vi "fotoncounter+lockin+fastratio_LV2010.vi"() -> ()   [LabVIEW 2010]
uses:
  Instance          14 40Saved   fotoncounter+lockin+fastratio v1 .vi
  Instance          13 40Saved   fotoncounter+lockin+fastratio v1 .vi
  Instance          33 40Saved   fotoncounter+lockin+fastratio v1 .vi
  Instance           2 40Saved   fotoncounter+lockin+fastratio v1 .vi
  Instance           5 40Saved   fotoncounter+lockin+fastratio v1 .vi
  Instance           6 40Saved   fotoncounter+lockin+fastratio v1 .vi
  Instance           7 40Saved   fotoncounter+lockin+fastratio v1 .vi
  Instance          15 40Saved   fotoncounter+lockin+fastratio v1 .vi
  Instance           8 40Saved   fotoncounter+lockin+fastratio v1 .vi
  Instance           9 40Saved   fotoncounter+lockin+fastratio v1 .vi
  Instance          10 40Saved   fotoncounter+lockin+fastratio v1 .vi
  Instance          11 40Saved   fotoncounter+lockin+fastratio v1 .vi
  Instance           1 40Saved   fotoncounter+lockin+fastratio v1 .vi
  Instance          18 40Saved   fotoncounter+lockin+fastratio v1 .vi
  Instance          19 40Saved   fotoncounter+lockin+fastratio v1 .vi
  Instance          23 40Saved   fotoncounter+lockin+fastratio v1 .vi
  Instance          17 40Saved   fotoncounter+lockin+fastratio v1 .vi
  Instance          22 40Saved   fotoncounter+lockin+fastratio v1 .vi
  Instance          20 40Saved   fotoncounter+lockin+fastratio v1 .vi
  Instance          21 40Saved   fotoncounter+lockin+fastratio v1 .vi
  Instance          26 40Saved   fotoncounter+lockin+fastratio v1 .vi
  Instance          27 40Saved   fotoncounter+lockin+fastratio v1 .vi
  Instance          29 40Saved   fotoncounter+lockin+fastratio v1 .vi
  <vilib>/Utility/file.llb/Write To Spreadsheet File (DBL).vi
  Instance          24 40Saved   fotoncounter+lockin+fastratio v1 .vi
  <vilib>/Utility/file.llb/Read From Spreadsheet File (DBL).vi
  Instance          32 40Saved   fotoncounter+lockin+fastratio v1 .vi
  Instance          31 40Saved   fotoncounter+lockin+fastratio v1 .vi
  Instance          30 40Saved   fotoncounter+lockin+fastratio v1 .vi
panel:
  out "lockin corrected count":cluster{dbl[], dbl[]}(graph)
  in  "Array":dbl[](array[numeric])
  in  "Lockin settings":T1={"slope"=1, "Input Mode"=0, "time constant"=6, "display type"=1, "Range"=7, "Line reject"=1, "Filter Type"=0, "Auto freq tuning"=TRUE, "Filter Frequency (Hz)"=1000.0, "Auto Sensitivity"=FALSE, "Auto Measure"=FALSE, "Auto Phase"=TRUE} {"Filter Frequency (Hz)" min=2.0 max=1250000.0 step=1.0; "Filter Type" items=["Flat", "Notch", "Low-Pass", "Bandpass"]; "Line reject" items=["OFF", "2F", "F", "F & 2F"]; "Range" items=["100 nV", "300 nV", "1 uV", "3 uV", "10 uV", "30 uV", "100 uV", "300 uV", "1 mV", "3 mV", "10 mV", "30 mV", "100 mV", "300 mV", "1 V", "3 V"]; "display type" items=["Output %", "Output calibrated ", "Ratio", "log Ratio", "ADC 1", "ADC 2", " ADC 3", "ADC 4", "Noise %", "Noise Calibrated", "Ref. Frequency"]; "time constant" items=["1 ms", "3 ms", "10 ms", "30 ms", "100 ms", "300 ms", "1 s", "3 s", "10 s", "30 s", "100 s", "300 s", "1 ks", "3 ks"]; "Input Mode" items=["Voltage Input ( A or A-B)", "Current Input 10E6 V/A", "Current Input 10E8 V/A"]; "slope" items=["6dB/octave", "12dB/octave"]}
  in  "Cluster":T2={"slope"=1, "Input Mode"=0, "time constant"=0, "display type"=1, "Range"=13} {"Range" items=["100 nV", "300 nV", "1 uV", "3 uV", "10 uV", "30 uV", "100 uV", "300 uV", "1 mV", "3 mV", "10 mV", "30 mV", "100 mV", "300 mV", "1 V", "3 V"]; "display type" items=["Output %", "Output calibrated ", "Ratio", "log Ratio", "ADC 1", "ADC 2", " ADC 3", "ADC 4", "Noise %", "Noise Calibrated", "Ref. Frequency"]; "time constant" items=["1 ms", "3 ms", "10 ms", "30 ms", "100 ms", "300 ms", "1 s", "3 s", "10 s", "30 s", "100 s", "300 s", "1 ks", "3 ks"]; "Input Mode" items=["Voltage Input ( A or A-B)", "Current Input 10E6 V/A", "Current Input 10E8 V/A"]; "slope" items=["6dB/octave", "12dB/octave"]}
  out "lockin":i32
  out "counter B":i32=147
  out "counter A":i32=5821
  out "LOCKIN OUTPUT DATA":cluster{"Y":dbl[], "Y":dbl[]}[](graph)=[{"Y"=[1.0], "Y"=[0.08234234]}]
  in  "EG&G 5209\nlockin amplifier\nGPIB address":u8=12 min=1 max=32 step=1
  out "# count periods done":i32=1
  out "Data Bit value":i32=1
  out "PHOTON COUNTER DATA":cluster{"all rows":dbl[], "all rows":dbl[]}[](graph)=[{"all rows"=[1.0], "all rows"=[5821.0]}, {"all rows"=[1.0], "all rows"=[147.0]}]
  in  "T select":i16(slide) scale=0.0..2.0
  in  "A scan step (V)":ext=-0.005 format="%.3e"
  in  "B scan step(V)":ext=-0.005 format="%.3e"
  in  "T scan step (V)":ext=0.02 format="%.3e"
  out "error 7":bool
  in  "A mode":bool=TRUE
  in  "B mode":bool=TRUE
  in  "T mode":bool=TRUE
  in  "A level (V)":ext=0.028 format="%.3e"
  in  "B level (V)":ext=0.028 format="%.3e"
  in  "T level (V)":ext=-0.01 format="%.3e"
  in  "B Preset":ext=1.0
  in  "count mode":i16(slide) scale=0.0..3.0 scale format="%.2f"
  in  "Path":path=path "C:/lvtemp/phototemp"
  out "error 6":bool
  in  "A slope":bool=TRUE
  in  "B slope":bool=TRUE
  in  "T slope":bool
  in  "trigger slope":bool
  out "error 5":bool
  in  "trigger level":ext=0.5 format="%.3f"
  in  "A scan step":ext=0.000005 format="%.3e"
  in  "dwell source":i32(slide) scale=0.0..1.0
  in  "dwell time":ext=0.1 format="%.4f"
  in  "# count periods\n(2000 max.)":i32=1
  in  "A select":i16(slide)=1 scale=0.0..1.0
  in  "B select":i16(slide)=1 scale=1.0..2.0 scale format="%.2f"
  in  "SR400\nphoton counter\nGPIB address":string="0:23"
  in  "B gate delay":ext=0.00027000000000000000001 format="%.3e"
  in  "B gate mode":i16(slide)=1 scale=0.0..2.0
  out "error 2":bool
  in  "B gate width":ext=0.00021 format="%.3e"
  in  "B scan step":ext=0.000005 format="%.3e"
  in  "A gate delay":ext=0.00001 format="%.3e"
  in  "A gate mode":i16(slide)=1 scale=0.0..2.0 scale format="%.2f"
  in  "A gate width":ext=0.00021 format="%.3e"
  in  "T Preset":ext=5.0
  # "SR400 PHOTON COUNTER + EG&G 5209 LOCKIN AMPLIFIER"
  # "ADDRESSING/TRIGGER/DWELL SETTINGS"
  # "COUNTER/INPUT SETTINGS"
  # "photon counter GPIB Board 0, address 23\nEG&G lockin GPIB Board 0, address 12"
  # "RISE\n\nFALL"
  # "(s)"
  # "note: valid dwell time\n0.002  to 60.0 s"
  # "(s)"
  # "DISCRIMINATOR SETTINGS"
  # "GATE SETTINGS"
  # "FIXED\n\nSCAN"
  # "RISE\n\nFALL"
  # "RISE\n\nFALL"
  # "FIXED\n\nSCAN"
  # "FIXED\n\nSCAN"
  # "RISE\n\nFALL"
  # "note: valid disc levels \n-0.30 to 0.30 V"
  # "note: valid scan steps \n-0.020 to 0.020 V"
  # "\"...The greatest trick the Devil ever pulled was convincing the world he didn't exist...\" (and then inventing LabView)..."
  # "This makes the lockin work again. no idea if the settings are right, or even need to be messed with"
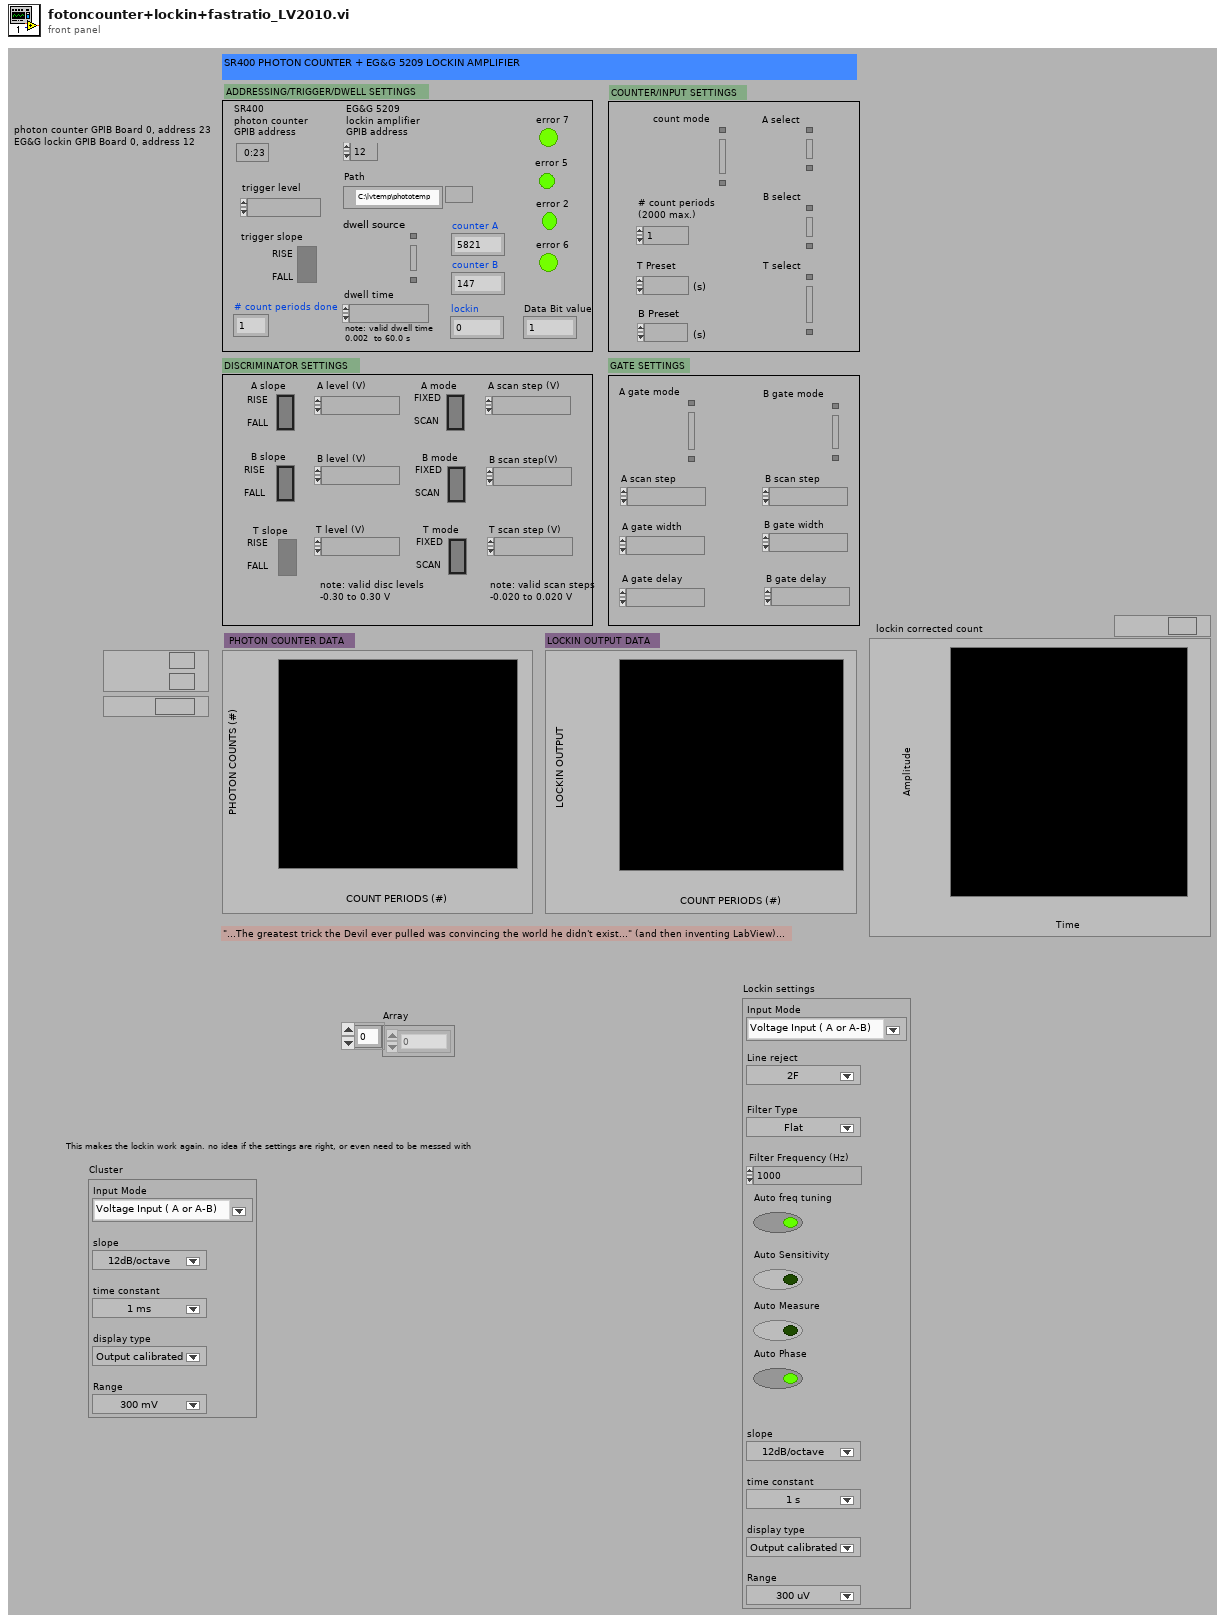
[diagram p1: front panel]
types:
  T1 = cluster{"slope":i32, "Input Mode":i32, "time constant":i32, "display type":i32, "Range":i32, "Line reject":i32, "Filter Type":i32, "Auto freq tuning":bool, "Filter Frequency (Hz)":dbl, "Auto Sensitivity":bool, "Auto Measure":bool, "Auto Phase":bool}
  T2 = cluster{"slope":i32, "Input Mode":i32, "time constant":i32, "display type":i32, "Range":i32}
  T3 = enum16{"open", "open or create", "create or replace", "create", "open (read only)"}
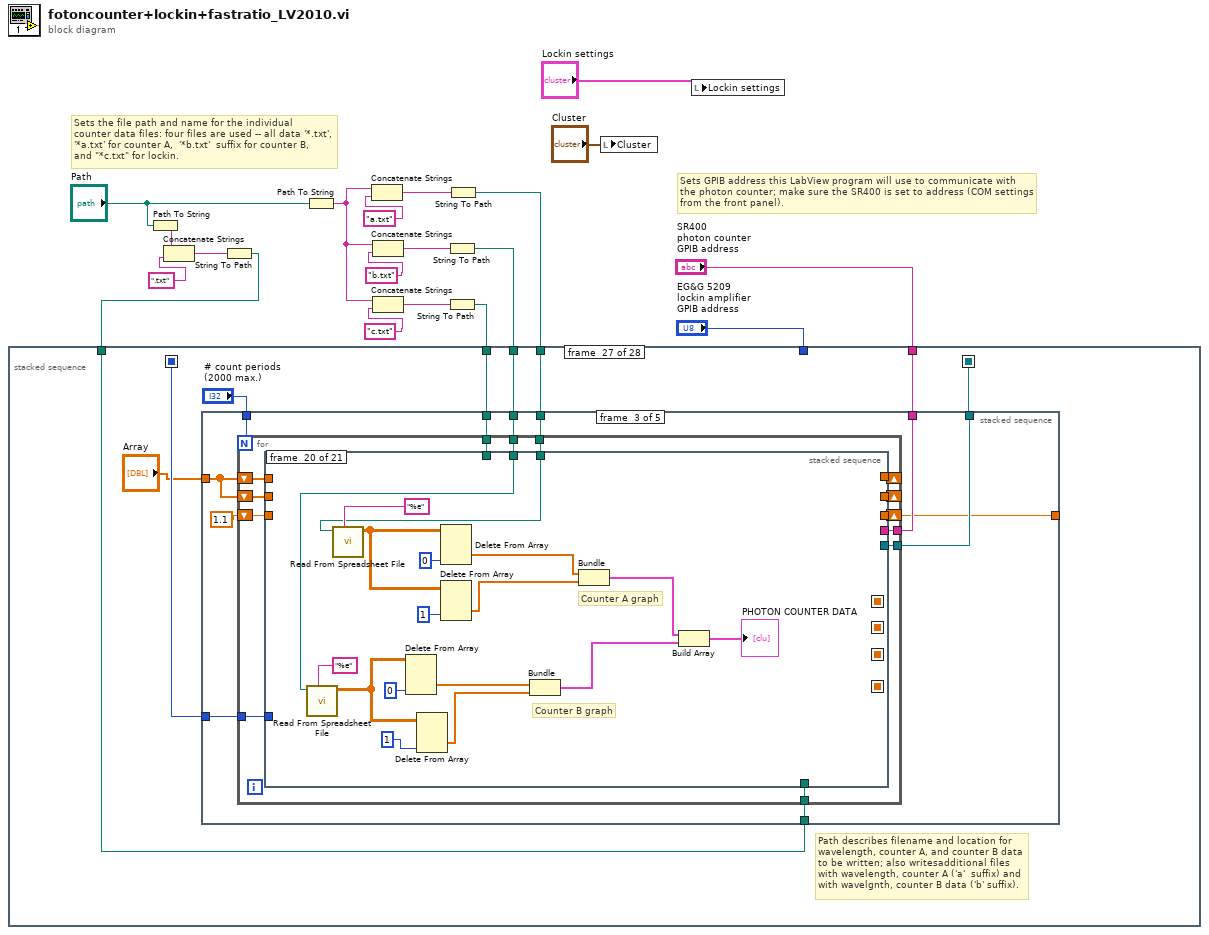
[diagram p0: block diagram]
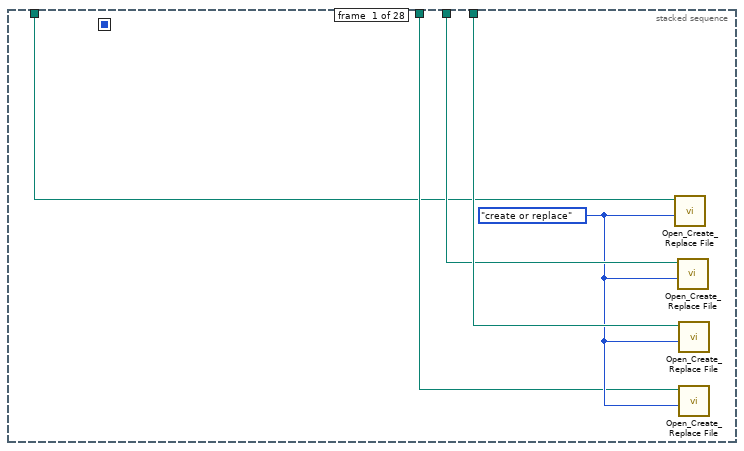
[diagram p2: hidden frame]
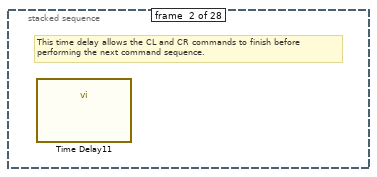
[diagram p3: hidden frame]
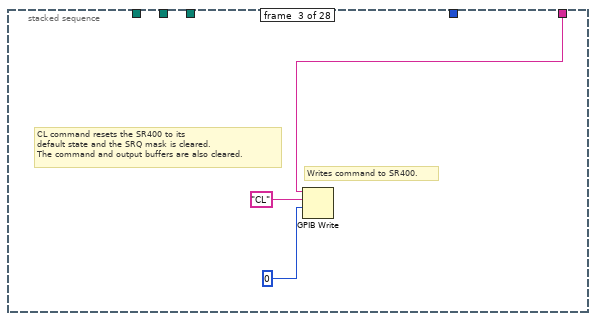
[diagram p4: hidden frame]
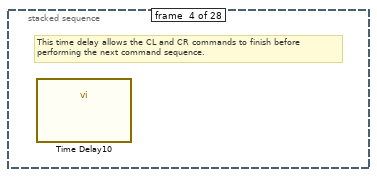
[diagram p5: hidden frame]
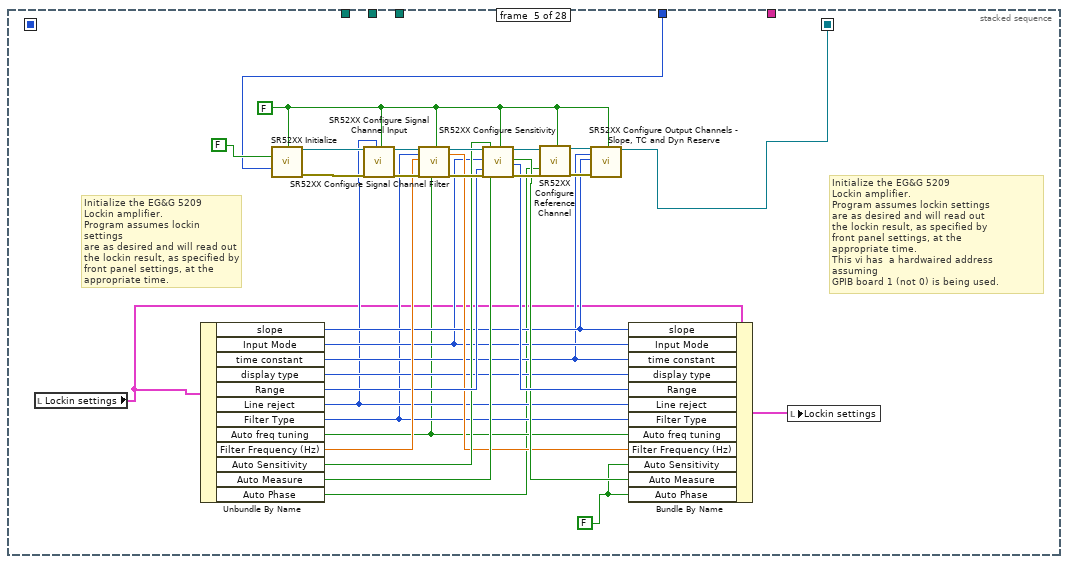
[diagram p6: hidden frame]
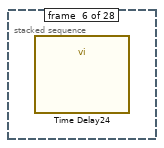
[diagram p7: hidden frame]
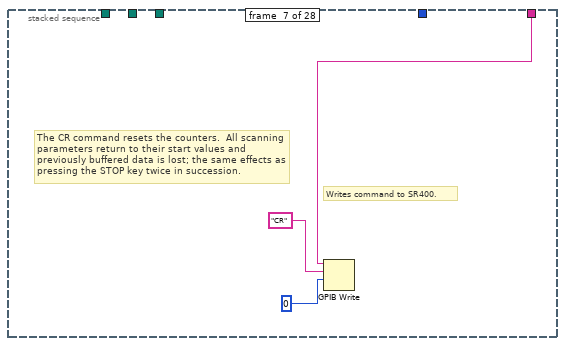
[diagram p8: hidden frame]
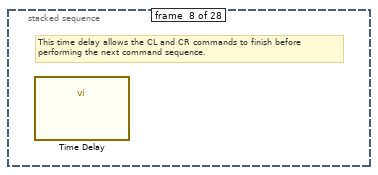
[diagram p9: hidden frame]
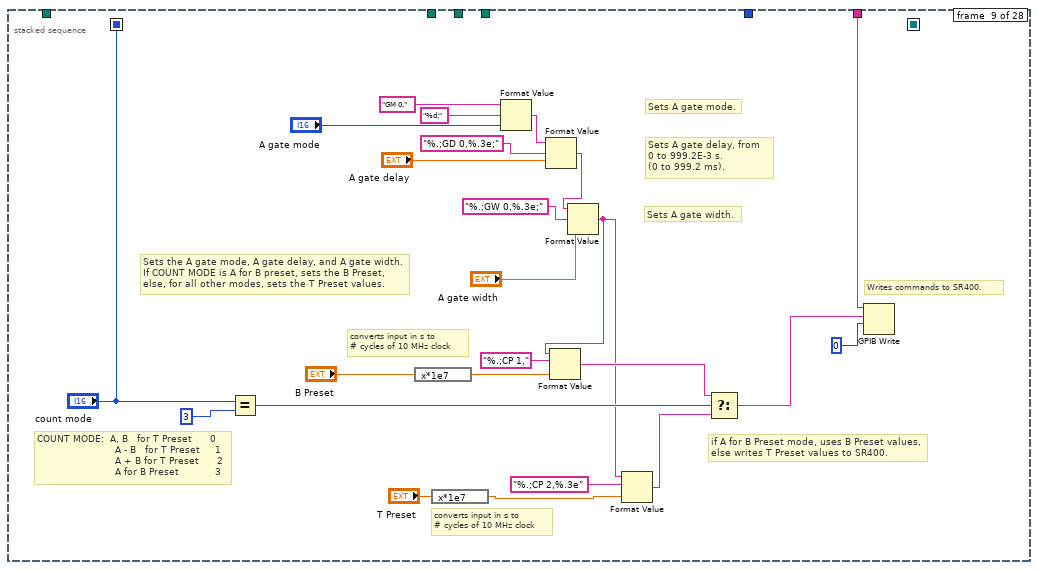
[diagram p10: hidden frame]
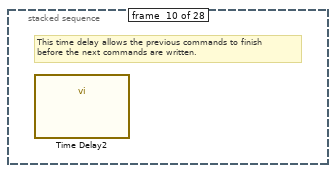
[diagram p11: hidden frame]
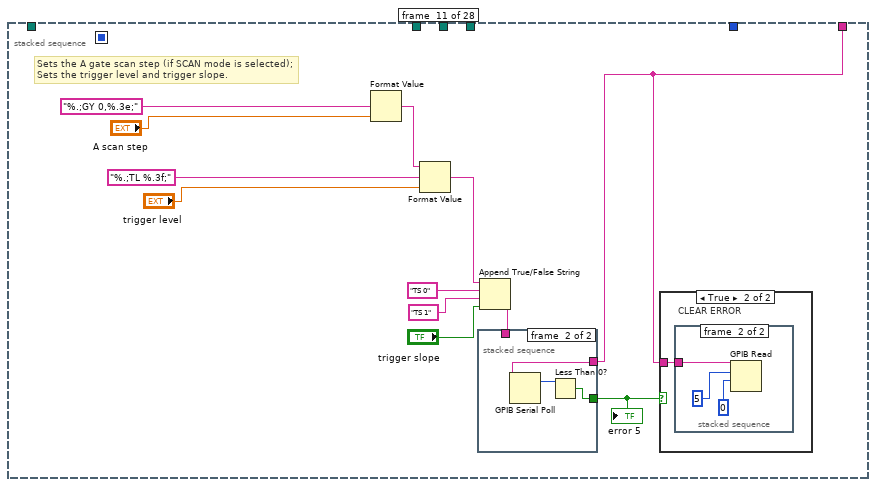
[diagram p12: hidden frame]
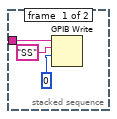
[diagram p14: hidden frame]
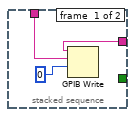
[diagram p15: hidden frame]
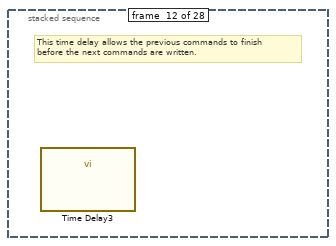
[diagram p16: hidden frame]
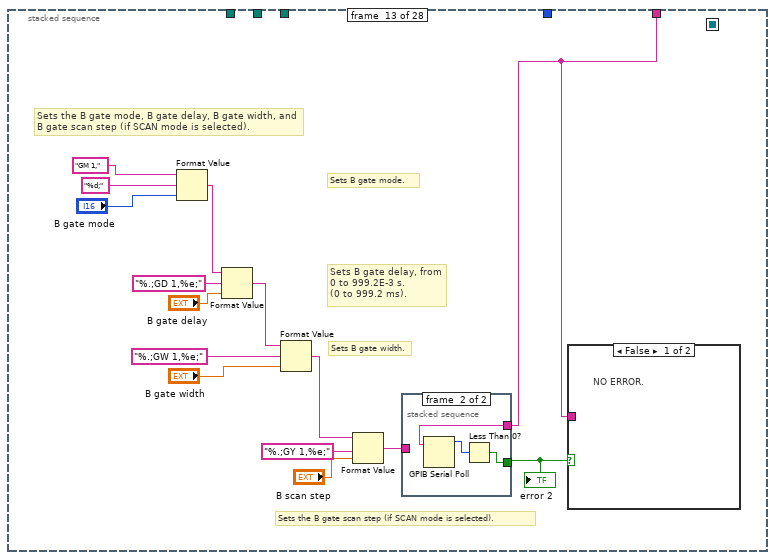
[diagram p17: hidden frame]
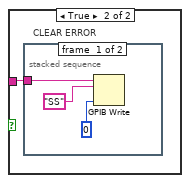
[diagram p18: hidden frame]
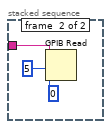
[diagram p19: hidden frame]
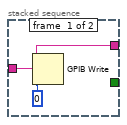
[diagram p20: hidden frame]
diagram:
  # "Sets the file path and name for the individual\ncounter data files: four files are used -- all data '*.txt',\n'*a.txt' for counter A,  '*b.txt'  suffix for counter B,\nand \"*c.txt\" for lockin."
  # "Sets GPIB address this LabView program will use to communicate with\nthe photon counter; make sure the SR400 is set to address (COM settings\nfrom the front panel)."
  n1 = Path To String(path="Path") -> (string=w13:string)
  n2 = Concatenate Strings(w13, ".txt") -> (w11:string)
  n3 = String To Path(string=w11) -> (path=w3:path)
  n4 = Path To String(path="Path") -> (string=w6:string)
  n5 = Concatenate Strings(w6, "a.txt") -> (w14:string)
  n6 = Concatenate Strings(w6, "b.txt") -> (w17:string)
  n7 = Concatenate Strings(w6, "c.txt") -> (w8:string)
  n8 = String To Path(string=w17) -> (path=w15:path)
  n9 = String To Path(string=w8) -> (path=w5:path)
  n10 = String To Path(string=w14) -> (path=w16:path)
  n11 = stacked-sequence {
    seq-local: [_ _ _ _ _ _ _ _ "count mode" _ _ _ _ _ _ _ _ _ _ _ _ _ _ _ _ _ _ _] -> [_ _ _ _ _ _ _ _ _ _ _ _ _ _ _ _ _ _ _ _ _ _ _ _ _ _ w221 _]
    seq-local: [_ _ _ _ w30 _ _ _ _ _ _ _ _ _ _ _ _ _ _ _ _ _ _ _ _ _ _ _] -> [_ _ _ _ _ _ _ _ _ _ _ _ _ _ _ _ _ _ _ _ _ _ _ _ _ _ w220 _]
    tunnel: "SR400\nphoton counter\nGPIB address" -> [_ _ w25 _ _ _ w60 _ w81 _ w87 _ w113 _ w142 _ w151 _ w157 _ w167 _ w187 _ w207 _ w227 _]
    tunnel: w16 -> [w24 _ _ _ _ _ _ _ _ _ _ _ _ _ _ _ _ _ _ _ _ _ _ _ _ _ w226 _]
    tunnel: w15 -> [w23 _ _ _ _ _ _ _ _ _ _ _ _ _ _ _ _ _ _ _ _ _ _ _ _ _ w225 _]
    tunnel: w3 -> [w20 _ _ _ _ _ _ _ _ _ _ _ _ _ _ _ _ _ _ _ _ _ _ _ _ _ w224 w392]
    tunnel: "EG&G 5209\nlockin amplifier\nGPIB address" -> [_ _ _ _ w31 _ _ _ _ _ _ _ _ _ _ _ _ _ _ _ _ _ _ _ _ _ _ _]
    tunnel: w5 -> [w21 _ _ _ _ _ _ _ _ _ _ _ _ _ _ _ _ _ _ _ _ _ _ _ _ _ w223 _]
    frame #0 {
      w22 = T3."create or replace" ("function (open:0)")
      n12 = call <vilib>:"Open_Create_Replace File.vi"("function (open:0)"=w22, "file path"=w20) -> ()  [unwired: 6 in, 4 out]
      n13 = call <vilib>:"Open_Create_Replace File.vi"("function (open:0)"=w22, "file path"=w23) -> ()  [unwired: 6 in, 4 out]
      n14 = call <vilib>:"Open_Create_Replace File.vi"("function (open:0)"=w22, "file path"=w24) -> ()  [unwired: 6 in, 4 out]
      n15 = call <vilib>:"Open_Create_Replace File.vi"("function (open:0)"=w22, "file path"=w21) -> ()  [unwired: 6 in, 4 out]
    }
    frame #1 {
      # "This time delay allows the CL and CR commands to finish before\nperforming the next command sequence."
      n16 = call "Time Delay11"() -> ()  [unwired: 11 in, 1 out]
    }
    frame #2 {
      # "Writes command to SR400."
      # "CL command resets the SR400 to its\ndefault state and the SRQ mask is cleared.\nThe command and output buffers are also cleared."
      n17 = GPIB Write(0:w25, 1:"CL", 2:0) -> ()  [unwired: 2 in, 2 out]
    }
    frame #3 {
      # "This time delay allows the CL and CR commands to finish before\nperforming the next command sequence."
      n18 = call "Time Delay10"() -> ()  [unwired: 11 in, 1 out]
    }
    frame #4 {
      w33 = FALSE ("reset")
      w49 = FALSE ("reset")
      # "Initialize the EG&G 5209\nLockin amplifier.\nProgram assumes lockin settings\nare as desired and will read out\nthe lockin result, as specified by \nfront panel settings, at the\nappropriate time."
      # "Initialize the EG&G 5209\nLockin amplifier.\nProgram assumes lockin settings\nare as desired and will read out\nthe lockin result, as specified by \nfront panel settings, at the\nappropriate time.\nThis vi has  a hardwaired address assuming \nGPIB board 1 (not 0) is being used."
      n19 = local read "Lockin settings"() -> (w29:T1)
      n20 = Unbundle By Name(w29) -> ("slope"=w41:i32, "Input Mode"=w40:i32, "time constant"=w39:i32, "display type"=w38:i32, "Range"=w47:i32, "Line reject"=w37:i32, "Filter Type"=w36:i32, "Auto freq tuning"=w35:bool, "Filter Frequency (Hz)"=w48:dbl, "Auto Sensitivity"=w45:bool, "Auto Measure"=w46:bool, "Auto Phase"=w34:bool)
      n21 = call "SR52XX Initialize"("Interface"=FALSE, "Port"=w31, "reset"=w49) -> ("VISA session"=w59:refnum<visa-resource-name>, "error out"=w58:errorcluster)  [unwired: 10 in, 1 out]
      n22 = call "SR52XX Configure Signal Channel Input"("VISA session (for class)"=w59, "error in (no error)"=w58, "Line Frequency Rejection Filter"=w37, "Update"=w49) -> ("VISA session"=w57:refnum<visa-resource-name>, "error out"=w55:errorcluster)  [unwired: 14 in]
      n23 = call "SR52XX Configure Signal Channel Filter"("VISA session (for class)"=w57, "FilterType"=w36, "Filter Frequency (Hz)"=w48, "error in (no error)"=w55, "Filter Tuning"=w35, "Update"=w49) -> ("VISA session"=w56:refnum<visa-resource-name>, "Filter Frequency (Hz) out"=w42:dbl, "error out"=w54:errorcluster)  [unwired: 11 in]
      n24 = call "SR52XX Configure Sensitivity"("VISA session (for class)"=w56, "Input Mode"=w40, "Range"=w47, "error in (no error)"=w54, "Auto Sensitivity"=w45, "Auto Measure"=w46, "Update"=w49) -> ("VISA session"=w53:refnum<visa-resource-name>, "Auto Measure out"=w43:bool, "Range Out"=w44:u8, "error out"=w52:errorcluster)  [unwired: 7 in, 2 out]
      n25 = call "SR52XX Configure Reference Channel"("VISA session (for class)"=w53, "Auto Phase"=w34, "error in (no error)"=w52, "Update"=w49) -> ("VISA session"=w51:refnum<visa-resource-name>, "error out"=w50:errorcluster)  [unwired: 12 in, 2 out]
      n26 = call "SR52XX Configure Output Channels - Slope, TC and Dyn Reserve"("VISA session (for class)"=w51, "Time Constant"=w39, "Slope"=w41, "error in (no error)"=w50, "Update"=w49) -> ("VISA session"=w30:refnum<visa-resource-name>)  [unwired: 11 in, 3 out]
      n27 = Bundle By Name(cluster=w29, "slope"=w41, "Input Mode"=w40, "time constant"=w39, "display type"=w38, "Range"=w44, "Line reject"=w37, "Filter Type"=w36, "Auto freq tuning"=w35, "Filter Frequency (Hz)"=w42, "Auto Sensitivity"=w33, "Auto Measure"=w43, "Auto Phase"=w33) -> (w28:T1)
      n28 = local write "Lockin settings"(w28) -> ()
    }
    frame #5 {
      n29 = call "Time Delay24"() -> ()  [unwired: 11 in, 1 out]
    }
    frame #6 {
      # "Writes command to SR400."
      # "The CR command resets the counters.  All scanning\nparameters return to their start values and \npreviously buffered data is lost; the same effects as\npressing the STOP key twice in succession."
      n30 = GPIB Write(0:w60, 1:"CR", 2:0) -> ()  [unwired: 2 in, 2 out]
    }
    frame #7 {
      # "This time delay allows the CL and CR commands to finish before\nperforming the next command sequence."
      n31 = call "Time Delay"() -> ()  [unwired: 11 in, 1 out]
    }
    frame #8 {
      # "if A for B Preset mode, uses B Preset values,\nelse writes T Preset values to SR400."
      # "converts input in s to\n# cycles of 10 MHz clock"
      # "converts input in s to\n# cycles of 10 MHz clock"
      # "Writes commands to SR400."
      # "Sets A gate delay, from \n0 to 999.2E-3 s.\n(0 to 999.2 ms)."
      # "Sets A gate width."
      # "Sets A gate mode."
      # "COUNT MODE:  A, B   for T Preset      0 \n                          A - B   for T Preset     1\n                          A + B for T Preset      2\n                          A for B Preset            3"
      # "Sets the A gate mode, A gate delay, and A gate width.\nIf COUNT MODE is A for B preset, sets the B Preset, \nelse, for all other modes, sets the T Preset values."
      n32 = Equal?(x="count mode", y=3) -> (x = y?=w73:bool)
      n33 = expression code="x*1e7"("B Preset") -> (w63:ext)
      n34 = expression code="x*1e7"("T Preset") -> (w65:ext)
      n35 = Format Value(string ("")="GM 0,", format string="%d;", value (0)="A gate mode") -> (output string=w80:string)
      n36 = Format Value(string ("")=w80, format string="%.;GD 0,%.3e;", value (0)="A gate delay") -> (output string=w77:string)
      n37 = Format Value(string ("")=w77, format string="%.;GW 0,%.3e;", value (0)="A gate width") -> (output string=w68:string)
      n38 = Format Value(string ("")=w68, format string="%.;CP 1,", value (0)=w63) -> (output string=w69:string)
      n39 = Format Value(string ("")=w68, format string="%.;CP 2,%.3e", value (0)=w65) -> (output string=w71:string)
      n40 = Select(t=w69, s=w73, f=w71) -> (s? t:f=w67:string)
      n41 = GPIB Write(0:w81, 1:w67, 2:0) -> ()  [unwired: 2 in, 2 out]
    }
    frame #9 {
      # "This time delay allows the previous commands to finish \nbefore the next commands are written."
      n42 = call "Time Delay2"() -> ()  [unwired: 11 in, 1 out]
    }
    frame #10 {
      # "Sets the A gate scan step (if SCAN mode is selected); \nSets the trigger level and trigger slope."
      n43 = Format Value(format string="%.;GY 0,%.3e;", value (0)="A scan step") -> (output string=w91:string)  [unwired: 1 in]
      n44 = Format Value(string ("")=w91, format string="%.;TL %.3f;", value (0)="trigger level") -> (output string=w94:string)
      n45 = Append True/False String(1:"trigger slope", 2:"TS 1", 3:"TS 0", 4:w94) -> (0:w98:string)
      n46 = stacked-sequence {
        tunnel: w87 -> [w107 w109]
        tunnel: w98 -> [w106 _]
        tunnel: [_ w111] -> w89
        frame #0 {
          n47 = GPIB Write(0:w107, 1:w106, 2:0) -> ()  [unwired: 2 in, 2 out]
        }
        frame #1 {
          n48 = GPIB Serial Poll(0:w109) -> (2:w110:i16)  [unwired: 1 in, 2 out]
          n49 = Less Than 0?(x=w110) -> (x < 0?=w111:bool)
        }
      }
      "error 5" <- w89
      n50 = case shown="True" w89 {
        tunnel: w87 -> [_ w99]
        frame False {
          # "NO ERROR."
        }
        frame True {
          # "CLEAR ERROR"
          n51 = stacked-sequence {
            tunnel: w99 -> [w100 w103]
            frame #0 {
              n52 = GPIB Write(0:w100, 1:"SS", 2:0) -> ()  [unwired: 2 in, 2 out]
            }
            frame #1 {
              n53 = GPIB Read(0:w103, 1:5, 2:0) -> ()  [unwired: 2 in, 3 out]
            }
          }
        }
      }
    }
    frame #11 {
      # "This time delay allows the previous commands to finish \nbefore the next commands are written."
      n54 = call "Time Delay3"() -> ()  [unwired: 11 in, 1 out]
    }
    frame #12 {
      # "Sets the B gate scan step (if SCAN mode is selected)."
      # "Sets B gate width."
      # "Sets B gate delay, from \n0 to 999.2E-3 s.\n(0 to 999.2 ms)."
      # "Sets B gate mode."
      # "Sets the B gate mode, B gate delay, B gate width, and \nB gate scan step (if SCAN mode is selected)."
      n55 = Format Value(string ("")="GM 1,", format string="%d;", value (0)="B gate mode") -> (output string=w118:string)
      n56 = Format Value(string ("")=w118, format string="%.;GD 1,%e;", value (0)="B gate delay") -> (output string=w112:string)
      n57 = Format Value(string ("")=w112, format string="%.;GW 1,%e;", value (0)="B gate width") -> (output string=w122:string)
      n58 = Format Value(string ("")=w122, format string="%.;GY 1,%e;", value (0)="B scan step") -> (output string=w125:string)
      n59 = stacked-sequence {
        tunnel: w113 -> [w134 w137]
        tunnel: [_ w139] -> w126
        tunnel: w125 -> [w136 _]
        frame #0 {
          n60 = GPIB Write(0:w134, 1:w136, 2:0) -> ()  [unwired: 2 in, 2 out]
        }
        frame #1 {
          n61 = GPIB Serial Poll(0:w137) -> (2:w138:i16)  [unwired: 1 in, 2 out]
          n62 = Less Than 0?(x=w138) -> (x < 0?=w139:bool)
        }
      }
      "error 2" <- w126
      n63 = case shown="False" w126 {
        tunnel: w113 -> [_ w127]
        frame False {
          # "NO ERROR."
        }
        frame True {
          # "CLEAR ERROR"
          n64 = stacked-sequence {
            tunnel: w127 -> [w128 w131]
            frame #0 {
              n65 = GPIB Write(0:w128, 1:"SS", 2:0) -> ()  [unwired: 2 in, 2 out]
            }
            frame #1 {
              n66 = GPIB Read(0:w131, 1:5, 2:0) -> ()  [unwired: 2 in, 3 out]
            }
          }
        }
      }
    }
    frame #13 {
      # "This time delay allows the previous commands to finish \nbefore the next commands are written."
      n67 = call "Time Delay4"() -> ()  [unwired: 11 in, 1 out]
    }
    frame #14 {
      # "Writes commands to SR400."
      # "Sets the input to counter A (INPUT1 or 10 MHz clock);\nSets the input to counter B (INPUT1 or INPUT2);"
      n68 = Format Value(string ("")="CI 0,", format string="%d;", value (0)="A select") -> (output string=w147:string)
      n69 = Format Value(string ("")=w147, format string="%.;CI 1,%d;", value (0)="B select") -> (output string=w140:string)
      n70 = GPIB Write(0:w142, 1:w140, 2:0) -> ()  [unwired: 2 in, 2 out]
    }
    frame #15 {
      # "This time delay allows the previous commands to finish \nbefore the next commands are written."
      n71 = call "Time Delay12"() -> ()  [unwired: 11 in, 1 out]
    }
    frame #16 {
      # "Writes commands to SR400."
      # "Sets the input to counter T (EXT TRIG, INPUT 2, or 10 MHz clock);"
      n72 = Pick Line(string ("")="CI 2,", multi-line string="0;\r2;\r3;", line index="T select") -> (output string=w150:string)
      n73 = GPIB Write(0:w151, 1:w150, 2:0) -> ()  [unwired: 2 in, 2 out]
    }
    frame #17 {
      # "This time delay allows the previous commands to finish \nbefore the next commands are written."
      n74 = call "Time Delay5"() -> ()  [unwired: 11 in, 1 out]
    }
    frame #18 {
      # "Writes commands to SR400."
      # "B counter discriminator level"
      # "T counter discriminator level"
      # "A counter discriminator level"
      # "Sets the A, B, and T discriminator levels.  \nThe input values must be between \n-0.3 V and 0.3 V (-300 mV and 300 mV)\nor else the counter leaves the default values\nof -0.01 V (-10 mV)."
      n75 = Format Value(string ("")="DL 0,", format string="%.4e;DL 1,", value (0)="A level (V)") -> (output string=w161:string)
      n76 = Format Value(string ("")=w161, format string="%.4e;DL 2,", value (0)="B level (V)") -> (output string=w162:string)
      n77 = Format Value(string ("")=w162, format string="%.4e;", value (0)="T level (V)") -> (output string=w155:string)
      n78 = GPIB Write(0:w157, 1:w155, 2:0) -> ()  [unwired: 2 in, 2 out]
    }
    frame #19 {
      # "This time delay allows the previous commands to finish \nbefore the next commands are written."
      n79 = call "Time Delay7"() -> ()  [unwired: 11 in, 1 out]
    }
    frame #20 {
      # "Sets the slope of the A, B, and T\ndiscriminator levels  (rise or fall)."
      n80 = Append True/False String(1:"A slope", 2:"DS 0,1;", 3:"DS 0,0;") -> (0:w174:string)  [unwired: 1 in]
      n81 = Append True/False String(1:"B slope", 2:"DS 1,1;", 3:"DS 1,0;", 4:w174) -> (0:w177:string)
      n82 = Append True/False String(1:"T slope", 2:"DS 2,1;", 3:"DS 2,0;", 4:w177) -> (0:w180:string)
      n83 = stacked-sequence {
        tunnel: w167 -> [w182 w186]
        tunnel: w180 -> [w183 _]
        tunnel: [_ w184] -> w170
        frame #0 {
          n84 = GPIB Write(0:w182, 1:w183, 2:0) -> ()  [unwired: 2 in, 2 out]
        }
        frame #1 {
          n85 = GPIB Serial Poll(0:w186) -> (2:w185:i16)  [unwired: 1 in, 2 out]
          n86 = Less Than 0?(x=w185) -> (x < 0?=w184:bool)
        }
      }
      "error 6" <- w170
    }
    frame #21 {
      # "This time delay allows the previous commands to finish \nbefore the next commands are written."
      n87 = call "Time Delay8"() -> ()  [unwired: 11 in, 1 out]
    }
    frame #22 {
      # "Sets the mode of the A, B, and T\ndiscriminators  (FIXED or SCAN)."
      n88 = Append True/False String(1:"A mode", 2:"DM 0,1;", 3:"DM 0,0;") -> (0:w194:string)  [unwired: 1 in]
      n89 = Append True/False String(1:"B mode", 2:"DM 1,1;", 3:"DM 1,0;", 4:w194) -> (0:w197:string)
      n90 = Append True/False String(1:"T mode", 2:"DM 2,1;", 3:"DM 2,0;", 4:w197) -> (0:w200:string)
      n91 = stacked-sequence {
        tunnel: w187 -> [w202 w206]
        tunnel: w200 -> [w203 _]
        tunnel: [_ w204] -> w190
        frame #0 {
          n92 = GPIB Write(0:w202, 1:w203, 2:0) -> ()  [unwired: 2 in, 2 out]
        }
        frame #1 {
          n93 = GPIB Serial Poll(0:w206) -> (2:w205:i16)  [unwired: 1 in, 2 out]
          n94 = Less Than 0?(x=w205) -> (x < 0?=w204:bool)
        }
      }
      "error 7" <- w190
    }
    frame #23 {
      # "This time delay allows the previous commands to finish \nbefore the next commands are written."
      n95 = call "Time Delay9"() -> ()  [unwired: 11 in, 1 out]
    }
    frame #24 {
      # "Writes commands to SR400."
      # "B  discriminator scan step"
      # "T  discriminator scan step"
      # "A discriminator scan step"
      # "Sets the A, B, and T discriminator \nscan step size.  The input values must be between \n-0.02 V and 0.02 V (-20 mV and 20 mV)."
      n96 = Format Value(string ("")="DY 0,", format string="%.4e;DY 1,", value (0)="A scan step (V)") -> (output string=w213:string)
      n97 = Format Value(string ("")=w213, format string="%.4e;DY 2,", value (0)="B scan step(V)") -> (output string=w214:string)
      n98 = Format Value(string ("")=w214, format string="%.4e;", value (0)="T scan step (V)") -> (output string=w208:string)
      n99 = GPIB Write(0:w207, 1:w208, 2:0) -> ()  [unwired: 2 in, 2 out]
    }
    frame #25 {
      # "This time delay allows the previous commands to finish \nbefore triggering the scan, taking the data, and reading\nout the buffer.."
      n100 = call "Time Delay6"() -> ()  [unwired: 11 in, 1 out]
    }
    frame #26 {
      # "Path describes filename and location for\nwavelength, counter A, and counter B data\nto be written; also writesadditional files\nwith wavelength, counter A ('a'  suffix) and\nwith wavelgnth, counter B data ('b' suffix)."
      n101 = stacked-sequence {
        tunnel: "# count periods\n(2000 max.)" -> [w232 _ w255 _ _]
        tunnel: w221 -> [w239 _ w251 _ _]
        tunnel: w227 -> [w230 w245 w252 w385 w388]
        tunnel: w226 -> [_ _ w256 _ _]
        tunnel: w225 -> [_ _ w253 _ _]
        tunnel: w224 -> [_ _ w254 _ _]
        tunnel: w220 -> [_ _ w249 _ _]
        tunnel: w223 -> [_ _ w250 _ _]
        tunnel: [_ _ w248 _ _] -> _
        tunnel: "Array" -> [_ _ w246 _ _]
        frame #0 {
          # "COUNT RESET (CR); \nSRQ AT END OF SCAN (SV 4); \n# PERIODS (NP);\n COUNT MODE: A,B FOR T (CM 0), \n                          A-B for T (CM 1), \n                          A+B for T (CM 2), \n                          A FOR B (CM 3);\nSet DWELL SOURCE and DWELL TIME;"
          # "Resets the counters; sets the count periods,\nthe count mode, dwell source and dwell time."
          n102 = Format Value(string ("")="CR;SV 4;", format string="NP %d;", value (0)=w232) -> (output string=w238:string)
          n103 = Pick Line(string ("")=w238, multi-line string="CM 0;\nCM 1;\n\rCM 2;\rCM 3;", line index=w239) -> (output string=w228:string)
          n104 = case shown="..0" "dwell source" {
            tunnel: ["dwell time" ext 0.0] -> w229
            frame ..0 {
            }
            frame 1.. {
              # "EXTERNAL"
            }
          }
          n105 = Format Value(string ("")=w228, format string="%.;DT %f", value (0)=w229) -> (output string=w236:string)
          n106 = GPIB Write(0:w230, 1:w236, 2:3) -> ()  [unwired: 2 in, 2 out]
        }
        frame #1 {
          # "Starts a new scan."
          n107 = GPIB Write(0:w245, 1:"CS", 2:3) -> ()  [unwired: 2 in, 2 out]
        }
        frame #2 {
          n108 = for {
            N: w255 -> [_]
            tunnel: w252 -> [w265]
            tunnel: w256 -> [w268]
            tunnel: w254 -> [w269]
            tunnel: w253 -> [w267]
            tunnel: w251 -> [w266]
            tunnel: w249 -> [w264]
            tunnel: w250 -> [w263]
            shift-right: [w262] -> w248
            shift-left: 1.1 -> [w261]
            shift-right: [w258] -> _
            shift-left: w246 -> [w260]
            shift-right: [w257] -> _
            shift-left: w246 -> [w259]
            n109 = stacked-sequence {
              seq-local: [_ _ _ w285 _ _ _ _ _ _ _ _ _ _ _ _ _ _ _ _ _] -> [_ _ _ _ _ _ _ w296 _ _ _ w311 _ _ _ w329 _ w346 _ _ _]
              seq-local: [_ _ _ _ _ _ _ w293 _ _ _ _ _ _ _ _ _ _ _ _ _] -> [_ _ _ _ _ _ _ _ _ _ _ _ _ _ _ _ _ w343 _ _ _]
              seq-local: [_ _ _ _ _ _ _ _ _ _ _ w308 _ _ _ _ _ _ _ _ _] -> [_ _ _ _ _ _ _ _ _ _ _ _ _ _ _ _ _ w342 _ _ _]
              seq-local: [_ _ _ _ _ _ _ _ _ _ _ _ _ w326 _ _ _ _ _ _ _] -> [_ _ _ _ _ _ _ _ _ _ _ _ _ _ _ w328 _ w335 _ _ _]
              tunnel: w269 -> [_ _ _ _ _ _ _ _ _ _ _ _ _ _ _ _ _ w352 _ _ _]
              tunnel: w268 -> [_ _ _ _ _ _ _ w295 _ _ _ _ _ _ _ _ _ _ _ w359 _]
              tunnel: w267 -> [_ _ _ _ _ _ _ _ _ _ _ w309 _ _ _ _ _ _ _ w372 _]
              tunnel: w266 -> [_ _ _ _ _ _ _ _ _ _ _ _ _ _ _ _ _ _ _ _ _]
              tunnel: w265 -> [w270 w282 _ w287 _ w290 _ w300 _ w305 _ w312 _ _ _ _ _ _ _ _ _]
              tunnel: w264 -> [_ _ _ _ _ _ _ _ _ _ _ _ _ w327 _ _ _ _ _ _ _]
              tunnel: w263 -> [_ _ _ _ _ _ _ _ _ _ _ _ _ _ _ w330 _ _ _ _ w375]
              tunnel: [_ _ _ _ _ _ _ _ _ _ _ _ _ _ _ _ _ w336 _ _ _] -> w262
              tunnel: w261 -> [_ _ _ _ _ _ _ _ _ _ _ _ _ _ _ _ _ w348 _ _ _]
              tunnel: w260 -> [_ _ _ _ _ _ _ _ _ _ _ _ _ _ _ _ _ w347 _ _ _]
              tunnel: w259 -> [_ _ _ _ _ _ _ _ _ _ _ _ _ _ _ _ _ w341 _ _ _]
              tunnel: [_ _ _ _ _ _ _ _ _ _ _ _ _ _ _ _ _ w338 _ _ _] -> w258
              tunnel: [_ _ _ _ _ _ _ _ _ _ _ _ _ _ _ _ _ w339 _ _ _] -> w257
              frame #0 {
                n110 = while {
                  tunnel: w270 -> [w272]
                  stop <- w271 stop-if-true
                  n111 = stacked-sequence {
                    tunnel: w272 -> [w273 _ w279 _]
                    tunnel: [_ _ w277 _] -> w271
                    frame #0 {
                      # "SS command reads the status bit: Bit 1\nindicates DATA READY, set at the end \nof each count period to indicate that counter\ndata is available."
                      # "Writes command to SR400;\nRead the status byte, bit 1;\nData Ready."
                      n112 = GPIB Write(0:w273, 1:"SS 1;", 2:3) -> ()  [unwired: 2 in, 2 out]
                    }
                    frame #1 {
                      n113 = call "Time Delay13"() -> ()  [unwired: 11 in, 1 out]
                    }
                    frame #2 {
                      # "GPIB command to read the value of \nthe status byte, bit 1 Data Ready."
                      n114 = GPIB Read(0:w279, 1:10, 2:0) -> (5:w278:string)  [unwired: 2 in, 2 out]
                      n115 = Decimal String To Number(string=w278) -> (number=w276:i32)  [unwired: 2 in, 1 out]
                      "Data Bit value" <- w276
                      n116 = Not Equal To 0?(x=w276) -> (x != 0?=w277:bool)
                    }
                    frame #3 {
                      n117 = call "Time Delay14"() -> ()  [unwired: 11 in, 1 out]
                    }
                  }
                }
              }
              frame #1 {
                # "Reads the scan position."
                n118 = GPIB Write(0:w282, 1:"NN", 2:3) -> ()  [unwired: 2 in, 2 out]
              }
              frame #2 {
                n119 = call "Time Delay20"() -> ()  [unwired: 11 in, 1 out]
              }
              frame #3 {
                # "GPIB command to read the scan position."
                n120 = GPIB Read(0:w287, 1:5, 2:3) -> (5:w286:string)  [unwired: 2 in, 2 out]
                n121 = Fract/Exp String To Number(string=w286) -> (number=w285:dbl)  [unwired: 3 in, 1 out]
                "# count periods done" <- w285
              }
              frame #4 {
                n122 = call "Time Delay15"() -> ()  [unwired: 11 in, 1 out]
              }
              frame #5 {
                # "Writes command to SR400\nto read the most recent complete\ndata point from counter A."
                n123 = GPIB Write(0:w290, 1:"QA", 2:3) -> ()  [unwired: 2 in, 2 out]
              }
              frame #6 {
                n124 = call "Time Delay18"() -> ()  [unwired: 11 in, 1 out]
              }
              frame #7 {
                # "FOR loop reads the A counter \ndata buffer, converts string to\na number, writes into an array; \nas well, appends data into the path\ngiven filename \"a\".txt; finally, \nwrites to spreadsheet file."
                # "READ CHANNEL A DATA."
                # "Sends A counter data to\nthe default file."
                # "Sends A counter data to file '*a.txt'"
                n125 = GPIB Read(0:w300, 1:20, 2:3) -> (5:w301:string)  [unwired: 2 in, 2 out]
                n126 = Fract/Exp String To Number(use system decimal point (T)=FALSE, string=w301) -> (number=w293:dbl)  [unwired: 2 in, 1 out]
                "counter A" <- w293
                n127 = Build Array(w296, w293) -> (w294:dbl[])
                n128 = Array To Spreadsheet String(array=w294, 3:"%e" ("format string")) -> (spreadsheet string=w297:string)  [unwired: 1 in]
                n129 = call <vilib>:"Write Characters To File.vi"("append to file? (new file:F)"=TRUE, "character string"=w297, "file path (dialog if empty)"=w295) -> ()  [unwired: 2 in, 1 out]
              }
              frame #8 {
                n130 = call "Time Delay16"() -> ()  [unwired: 11 in, 1 out]
              }
              frame #9 {
                # "Writes command to SR400\nto read the most recent complete\ndata point from counter B."
                n131 = GPIB Write(0:w305, 1:"QB", 2:3) -> ()  [unwired: 2 in, 2 out]
              }
              frame #10 {
                n132 = call "Time Delay17"() -> ()  [unwired: 11 in, 1 out]
              }
              frame #11 {
                # "B counter data"
                # "count period #"
                # "B counter data read: Same \nprocedure as for the A counter.  \nAs well, for mode \nA for B, no data to read."
                # "READ CHANNEL B DATA."
                # "Sends B counter data to file '*b.txt'"
                n133 = GPIB Read(0:w312, 1:20, 2:3) -> (5:w316:string)  [unwired: 2 in, 2 out]
                n134 = Fract/Exp String To Number(use system decimal point (T)=FALSE, string=w316) -> (number=w308:dbl)  [unwired: 2 in, 1 out]
                "counter B" <- w308
                n135 = Build Array(w311, w308) -> (w310:dbl[])
                n136 = Array To Spreadsheet String(array=w310, 3:"%e" ("format string")) -> (spreadsheet string=w313:string)  [unwired: 1 in]
                n137 = call <vilib>:"Write Characters To File.vi"("append to file? (new file:F)"=TRUE, "character string"=w313, "file path (dialog if empty)"=w309) -> ()  [unwired: 2 in, 1 out]
              }
              frame #12 {
                n138 = call "Time Delay19"() -> ()  [unwired: 11 in, 1 out]
              }
              frame #13 {
                # "Read Lockin Output"
                n139 = local read "Lockin settings"() -> (w325:T1)
                n140 = Unbundle By Name(w325) -> ("slope"=w324:i32, "Input Mode"=w323:i32, "time constant"=w322:i32, "display type"=w321:i32, "Range"=w320:i32)
                n141 = call "SR5209 Read Output"("VISA session (for class)"=w327, "Input Mode"=w323, "Time Constant"=w322, "Display Type"=w321, "Range"=w320, "Slope"=w324) -> ("Output (FP)"=w326:dbl)  [unwired: 5 in, 8 out]
                "lockin" <- w326
              }
              frame #14 {
                n142 = call "Time Delay22"() -> ()  [unwired: 11 in, 1 out]
              }
              frame #15 {
                # "lockin data"
                # "count period #"
                # "Sends lockin data to file '*c.txt'"
                n143 = Build Array(w329, w328) -> (w331:dbl[])
                n144 = Array To Spreadsheet String(array=w331, 3:"%e" ("format string")) -> (spreadsheet string=w332:string)  [unwired: 1 in]
                n145 = call <vilib>:"Write Characters To File.vi"("append to file? (new file:F)"=TRUE, "character string"=w332, "file path (dialog if empty)"=w330) -> ()  [unwired: 2 in, 1 out]
              }
              frame #16 {
                n146 = call "Time Delay23"() -> ()  [unwired: 11 in, 1 out]
              }
              frame #17 {
                # "lockin data"
                # "B counter data"
                # "A counter data"
                # "count period #"
                # "WRITE CHANNEL A, B DATA, and lockin data to default file."
                # "Sends count period #,\nA counter, B counter data,\nand lockin output \nto the default file."
                n147 = Greater?(x=w348, y=1) -> (0:w350:bool)
                n148 = Subtract(x=w343, y=w342) -> (x-y=w345:dbl)
                n149 = case shown="False" w350 {
                  tunnel: w335 -> [_ w357]
                  tunnel: w348 -> [w356 _]
                  tunnel: [w356 w357] -> w336
                  frame False {
                  }
                  frame True {
                  }
                }
                n150 = Multiply(x=w345, y=w336) -> (x*y=w344:dbl)
                n151 = Divide(x=w344, y=w335) -> (x/y=w340:dbl)
                n152 = Build Array (concatenate)(w341, w340) -> (w339:dbl[])
                n153 = Build Array(w346, w343, w342, w335) -> (w353:dbl[])
                n154 = call-poly <vilib>:"Write To Spreadsheet File.vi"("transpose? (no:F)"=FALSE, "format (%.3f)"="%.10e" ("format string"), "append to file? (new file:F)"=TRUE, "1D data"=w353, "file path (dialog if empty)"=w352) -> ()  [unwired: 3 in, 1 out]
                n155 = Build Array (concatenate)(w347, w346) -> (w338:dbl[])
                n156 = Bundle(w338, w339) -> (→"lockin corrected count":cluster{dbl[], dbl[]})  [unwired: 1 in]
              }
              frame #18 {
                n157 = call "Time Delay21"() -> ()  [unwired: 11 in, 1 out]
              }
              frame #19 {
                # "Counter B graph"
                # "Counter A graph"
                n158 = call-poly <vilib>:"Read From Spreadsheet File.vi"("format (%.3f)"="%e", "file path (dialog if empty)"=w372) -> ("all rows"=w362:dbl[][])  [unwired: 5 in, 4 out]
                n159 = call-poly <vilib>:"Read From Spreadsheet File.vi"("format (%.3f)"="%e", "file path (dialog if empty)"=w359) -> ("all rows"=w367:dbl[][])  [unwired: 5 in, 4 out]
                n160 = Delete From Array(array=w362, index (col)=0 ("disabled index (col)")) -> (deleted portion=w363:dbl[])  [unwired: 2 in, 1 out]
                n161 = Delete From Array(array=w362, index (col)=1 ("disabled index (col)")) -> (deleted portion=w364:dbl[])  [unwired: 2 in, 1 out]
                n162 = Delete From Array(array=w367, index (col)=0 ("disabled index (col)")) -> (deleted portion=w369:dbl[])  [unwired: 2 in, 1 out]
                n163 = Delete From Array(array=w367, index (col)=1 ("disabled index (col)")) -> (deleted portion=w368:dbl[])  [unwired: 2 in, 1 out]
                n164 = Bundle "Bundle"("all rows"=w363, "all rows"=w364) -> (w360:cluster{"all rows":dbl[], "all rows":dbl[]})  [unwired: 1 in]
                n165 = Bundle "Bundle"("all rows"=w369, "all rows"=w368) -> (w361:cluster{"all rows":dbl[], "all rows":dbl[]})  [unwired: 1 in]
                n166 = Build Array(w361, w360) -> (→"PHOTON COUNTER DATA":cluster{"all rows":dbl[], "all rows":dbl[]}[])
              }
              frame #20 {
                # "Send to Graph"
                # "Lockin graph"
                n167 = call-poly <vilib>:"Read From Spreadsheet File.vi"("format (%.3f)"="%e", "file path (dialog if empty)"=w375) -> ("all rows"=w382:dbl[][])  [unwired: 5 in, 4 out]
                n168 = Delete From Array(array=w382, index (col)=0 ("disabled index (col)")) -> (deleted portion=w377:dbl[])  [unwired: 2 in, 1 out]
                n169 = Delete From Array(array=w382, index (col)=1 ("disabled index (col)")) -> (deleted portion=w376:dbl[])  [unwired: 2 in, 1 out]
                n170 = call "Convert to Dynamic Data"("Array"=w377) -> ("Dynamic Data Type"=w379:dynamicdata)  [unwired: 3 in]
                n171 = call "Convert to Dynamic Data2"("Array"=w376) -> ("Dynamic Data Type"=w378:dynamicdata)  [unwired: 3 in]
                n172 = call "Build XY Graph"("Y Input"=w378, "X Input"=w379) -> ("XY Graph"=→"LOCKIN OUTPUT DATA":cluster{"Y":dbl[], "Y":dbl[]}[])  [unwired: 8 in, 1 out]
              }
            }
          }
        }
        frame #3 {
          # "CLEAR STATUS BYTE, SEND STATUS."
          n173 = GPIB Write(0:w385, 1:"SS", 2:3) -> ()  [unwired: 2 in, 2 out]
        }
        frame #4 {
          # "CLEAR STATUS."
          n174 = GPIB Read(0:w388, 1:6, 2:0) -> ()  [unwired: 2 in, 3 out]
        }
      }
    }
    frame #27 {
      # "Save the data to a file and location\nspecified by the user."
      n175 = Two Button Dialog(message="Would you like to save the graph?", 1:"Don't Save" ("F button name (\"Cancel\")"), 2:"Save" ("T button name (\"OK\")")) -> (T button?=w391:bool)
      n176 = case shown="True" w391 {
        tunnel: w392 -> [_ w396]
        frame False {
        }
        frame True {
          n177 = stacked-sequence {
            seq-local: [w398 _] -> [_ w400]
            tunnel: w396 -> [w397 _]
            frame #0 {
              n178 = call-poly <vilib>:"Read From Spreadsheet File.vi"("format (%.3f)"="%e", "file path (dialog if empty)"=w397) -> ("all rows"=w398:dbl[][])  [unwired: 5 in, 4 out]
            }
            frame #1 {
              n179 = call-poly <vilib>:"Write To Spreadsheet File.vi"("format (%.3f)"="%e", "2D data"=w400) -> ()  [unwired: 6 in, 1 out]
            }
          }
        }
      }
    }
  }
  n180 = local write "Cluster"("Cluster") -> ()
  n181 = local write "Lockin settings"("Lockin settings") -> ()
